vi "Configure Measurement Function.vi"(5 "Enable Resistance Measurement (F: Disable)":bool, 6 "Enable Voltage Measurement (F: Disable)":bool, 7 "Enable Current Measurement (T: Enable)":bool=TRUE, 8 "error in (no error)":errorcluster, 9 "Enable Charge Measurement (F: Disable)":bool, 10 "Channel (1: Channel 1)":i32(ring)=1 items=["Channel 1"=1, "Channel 2"=2], 11 "VISA resource name":refnum<visa-resource-name>) -> (0 "error out":errorcluster, 3 "VISA resource name out":refnum<visa-resource-name>)   [LabVIEW 2017, in "Keysight B2980 Series.lvlib"]
doc: "Enables the specified measurement functions."
uses:
  Keysight B2980 Series.lvlib
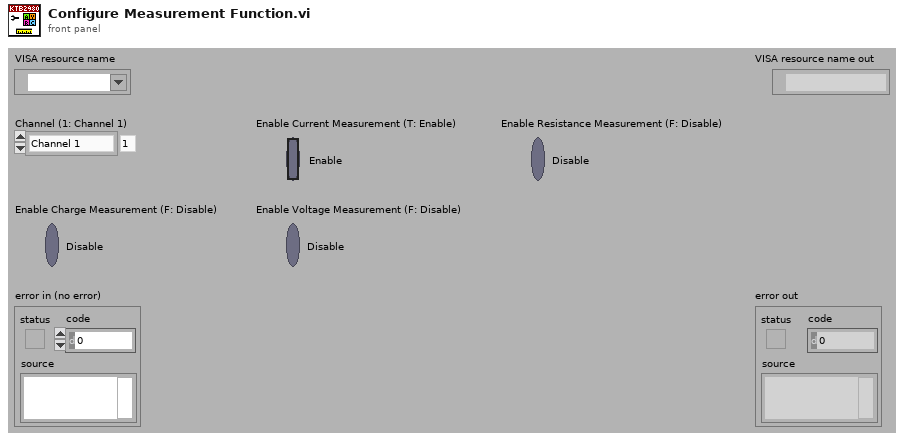
[diagram p1: front panel]
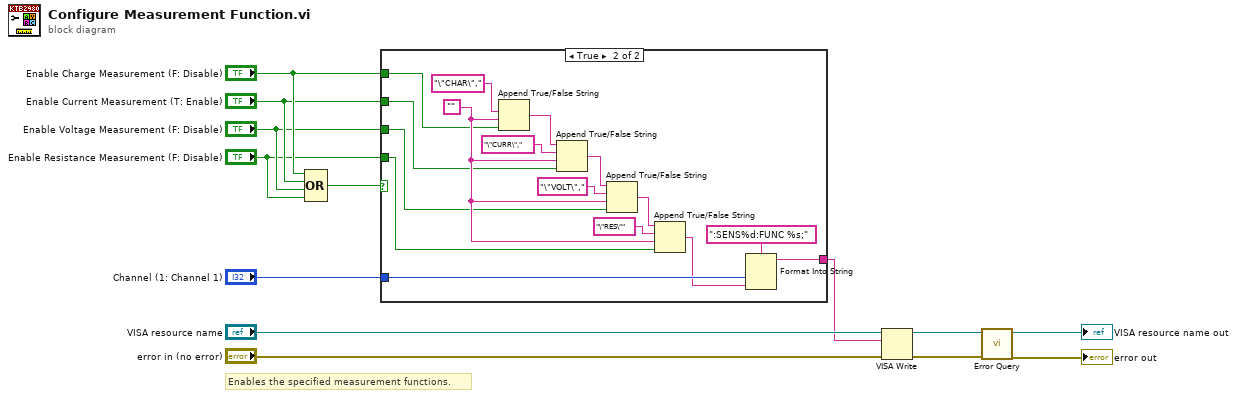
[diagram p0: block diagram]
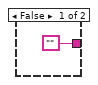
[diagram p2: hidden frame]
diagram:
  # "Enables the specified measurement functions."
  n1 = Compound Arithmetic op=OR("Enable Charge Measurement (F: Disable)", "Enable Current Measurement (T: Enable)", "Enable Voltage Measurement (F: Disable)", "Enable Resistance Measurement (F: Disable)") -> (w5:bool)
  n2 = case shown="True" w5 {
    tunnel: "Channel (1: Channel 1)" -> [_ w21]
    tunnel: ["" w19] -> w6
    tunnel: "Enable Charge Measurement (F: Disable)" -> [_ w15]
    tunnel: "Enable Current Measurement (T: Enable)" -> [_ w16]
    tunnel: "Enable Voltage Measurement (F: Disable)" -> [_ w17]
    tunnel: "Enable Resistance Measurement (F: Disable)" -> [_ w18]
    frame False {
    }
    frame True {
      w23 = ""
      n3 = Append True/False String(1:w15, 2:w23, 3:"\"CHAR\"," ("true string")) -> (0:w30:string)  [unwired: 1 out]
      n4 = Append True/False String(1:w16, 2:w23, 3:"\"CURR\"," ("true string"), 4:w30) -> (0:w29:string)
      n5 = Append True/False String(1:w17, 2:w23, 3:"\"VOLT\"," ("true string"), 4:w29) -> (0:w28:string)
      n6 = Append True/False String(1:w18, 2:w23, 3:"\"RES\"" ("true string"), 4:w28) -> (0:w20:string)
      n7 = Format Into String(format string=":SENS%d:FUNC %s;", w21, w20) -> (resulting string=w19:string)  [unwired: 2 in, 1 out]
    }
  }
  n8 = VISA Write(VISA resource name="VISA resource name", write buffer=w6, error in (no error)="error in (no error)") -> (VISA resource name out=w11:refnum<visa-resource-name>, error out=w10:errorcluster)  [unwired: 1 out]
  n9 = call "Error Query.vi"("error in (no error)"=w10, "VISA resource name"=w11) -> ("error out"=→"error out":errorcluster, "VISA resource name out"=→"VISA resource name out":refnum<visa-resource-name>)  [unwired: 8 out]
